vi "Create Commands.vi"(5 "Sequencer":refnum<class "MessageQ.lvclass">, 6 "Variables":refnum<class "Variables.lvclass">, 7 "VolatusAPI":refnum<class "VolatusAPI.lvclass">, 8 "error in (no error)":refnum<class "MultiErrors.lvclass">, 10 "Command Config":refnum<class "Command Config.lvclass">) -> (0 "error out":refnum<class "MultiErrors.lvclass">, 3 "Command":T1)   [LabVIEW 2023, in "VolatusSeq.lvlib" / "State.lvclass"]
uses:
  State.lvclass
  VolatusErrorUtilities/MultiErrors/MultiErrors.lvclass
  VolatusSeqConfig/Command Config/Command Config.lvclass
  Volatus/VolatusAPI/VolatusAPI.lvclass
  Command.ctl
  Volatus/MessageQ/MessageQ.lvclass
  Format String/Format String.lvclass
  VolatusSeqConfig/Command Type.ctl
  messages/CmdDigital/Data.ctl
  messages/CmdAnalog/Data.ctl
  Send Type.ctl
  lv-vecto/Vecto/Channel DBL/Channel DBL.lvclass
  Variables/Variables.lvclass
  VolatusSeqConfig/Digital Command Config/Digital Command Config.lvclass
  VolatusSeqConfig/Numeric Command Config/Numeric Command Config.lvclass
  VolatusSeqConfig/Transition Command Config/Transition Command Config.lvclass
  VolatusSeqConfig/Start Log Command Config/Start Log Command Config.lvclass
  VolatusSeqConfig/Start Seq Command Config/Start Seq Command Config.lvclass
  VolatusSeqConfig/Event Command Config/Event Command Config.lvclass
  VolatusSeqConfig/Error Command Config/Error Command Config.lvclass
  VolatusSeqConfig/HTTP Command Config/HTTP Command Config.lvclass
  VolatusSeqConfig/Reset Var Command Config/Reset Var Command Config.lvclass
  Variables/Variables.lvclass/Variables.ctl
  VolatusSeqConfig/Inc Var Command Config/Inc Var Command Config.lvclass
  VolatusSeqConfig/Dec Var Command Config/Dec Var Command Config.lvclass
  VolatusSeqConfig/Save Var Command Config/Save Var Command Config.lvclass
  VolatusSeqConfig/Load Var Command Config/Load Var Command Config.lvclass
  VolatusSeqConfig/Set Var Command Config/Set Var Command Config.lvclass
  VolatusSeqConfig/Add To Var Command Config/Add To Var Command Config.lvclass
  State.lvclass/State.ctl
  VolatusSeqConfig/VolatusSeqConfig.lvlib
  messages/CmdDigital/CmdDigital.lvlib
  messages/CmdAnalog/CmdAnalog.lvlib
  VolatusSeq.lvlib
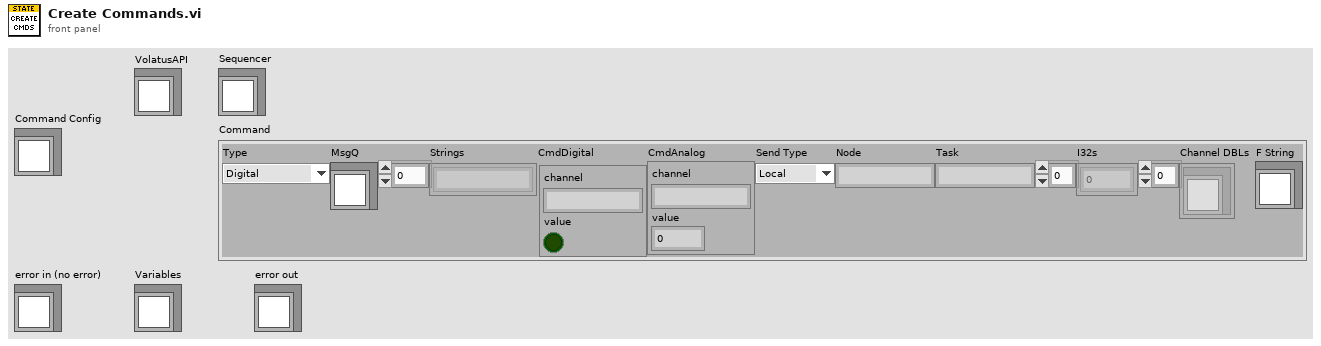
[diagram p1: front panel]
types:
  T1 = typedef "VolatusSeq.lvlib/Command.ctl" = cluster{"Type":T2, "MsgQ":refnum<class "MessageQ.lvclass">, "Strings":string[], "CmdDigital":T3, "CmdAnalog":T4, "Send Type":T5, "Node":string, "Task":string, "I32s":i32[], "Channel DBLs":refnum<class "Channel DBL.lvclass">[], "F String":refnum<class "Format String.lvclass">}
  T2 = typedef "VolatusSeqConfig.lvlib/Command Type.ctl" = enum16{"Digital", "Numeric", "Transition", "Stop", "StartLog", "StopLog", "Start", "Event", "Error", "HTTP", "ResetVar", "IncVar", "DecVar", "SaveVar", "LoadVar", "AddVar", "SubVar", "SetVar", "AddToVar"}
  T3 = typedef "CmdDigital.lvlib/Data.ctl" = cluster{"channel":string, "value":bool}
  T4 = typedef "CmdAnalog.lvlib/Data.ctl" = cluster{"channel":string, "value":dbl}
  T5 = typedef "VolatusSeq.lvlib/Send Type.ctl" = enum16{"Local", "Remote"}
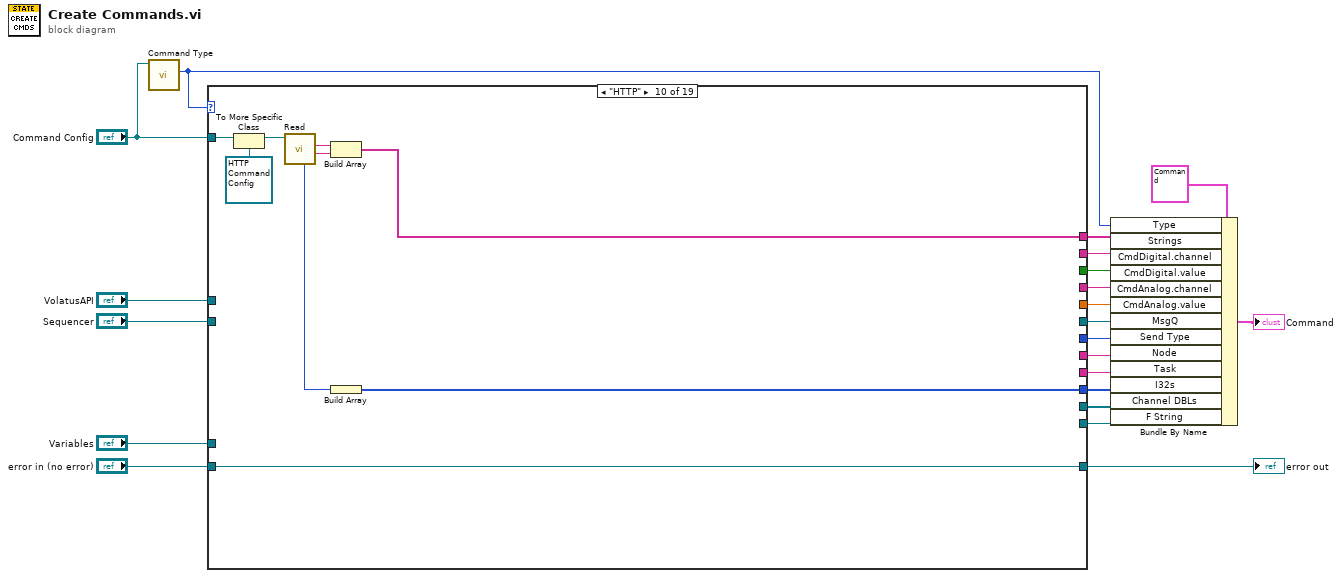
[diagram p0: block diagram]
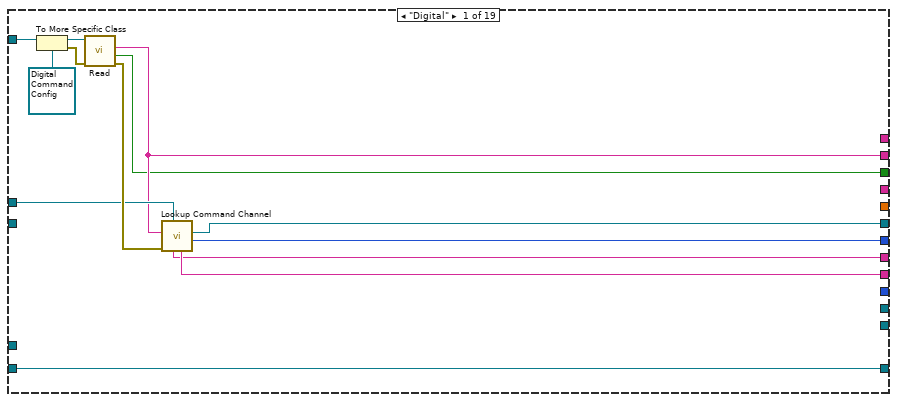
[diagram p2: hidden frame]
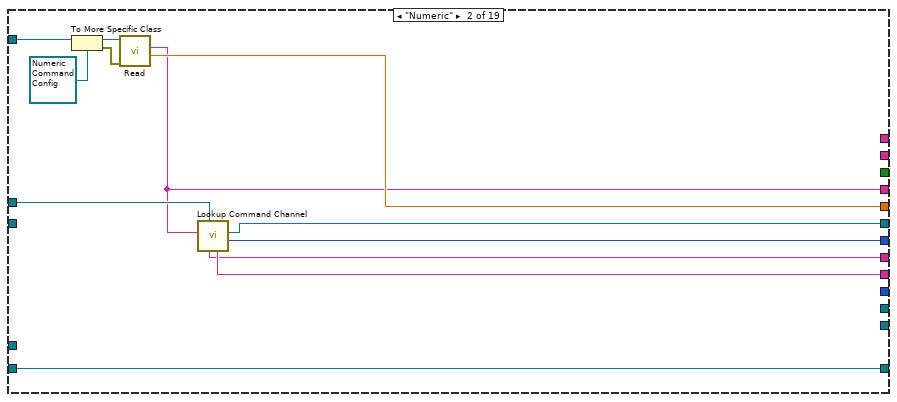
[diagram p3: hidden frame]
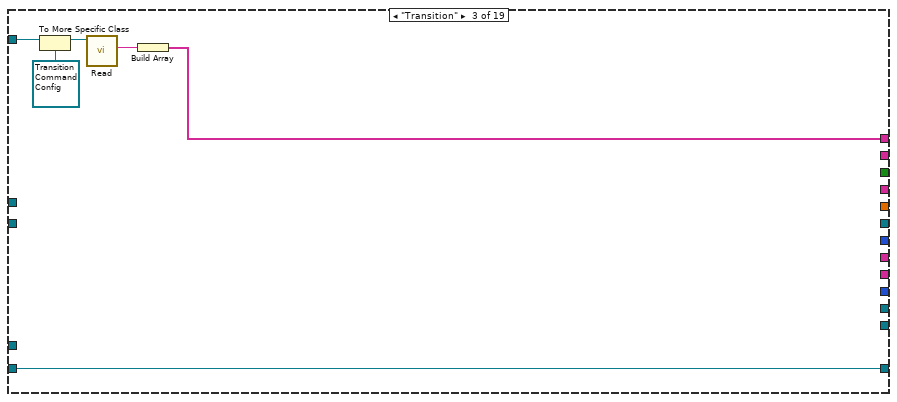
[diagram p4: hidden frame]
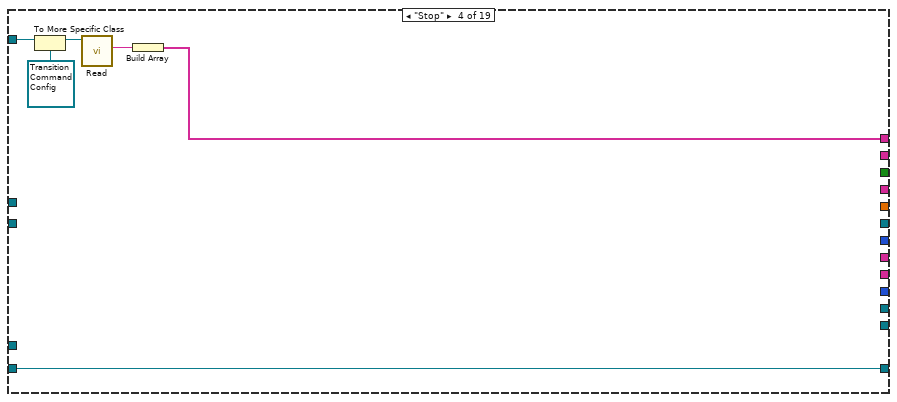
[diagram p5: hidden frame]
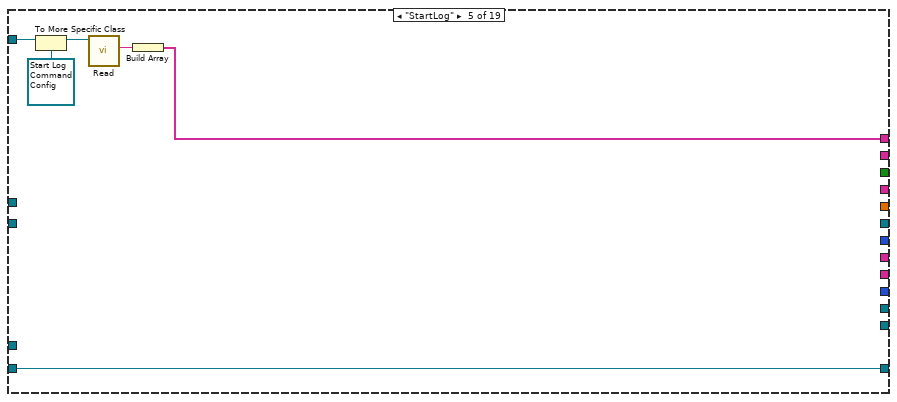
[diagram p6: hidden frame]
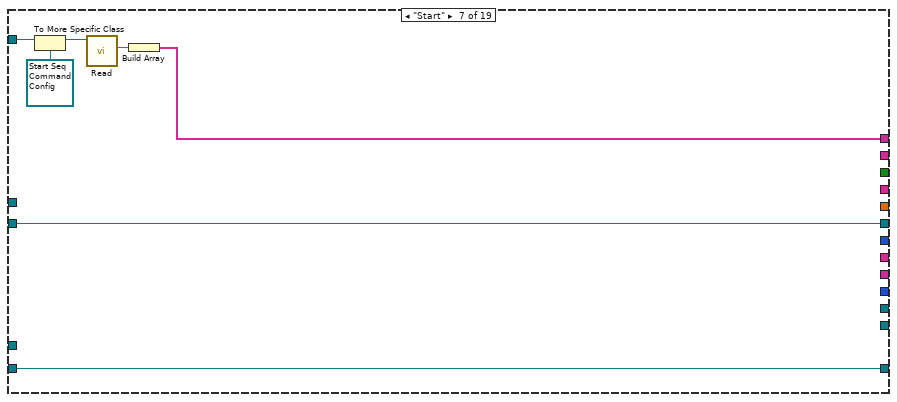
[diagram p8: hidden frame]
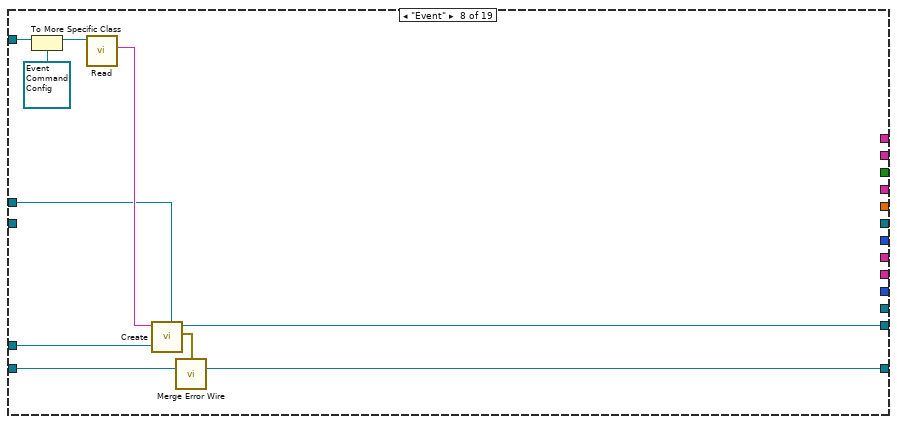
[diagram p9: hidden frame]
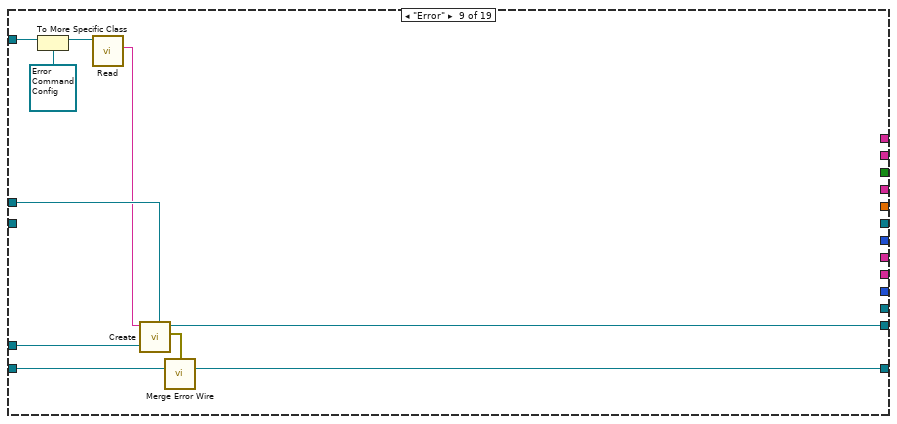
[diagram p10: hidden frame]
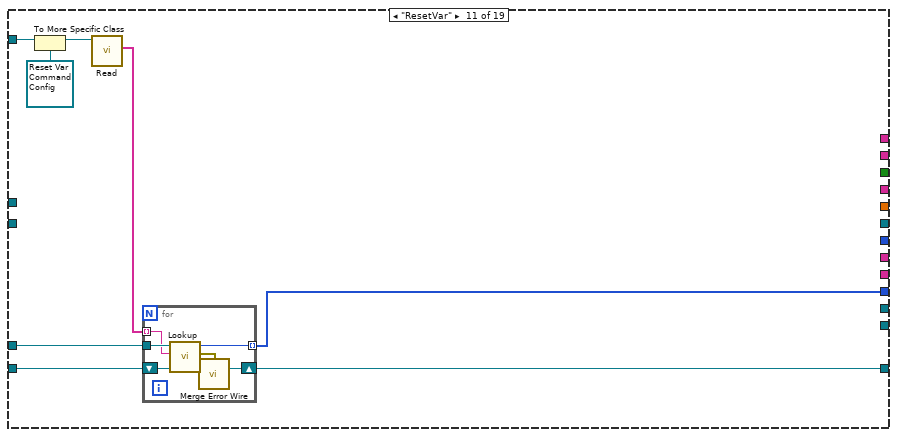
[diagram p11: hidden frame]
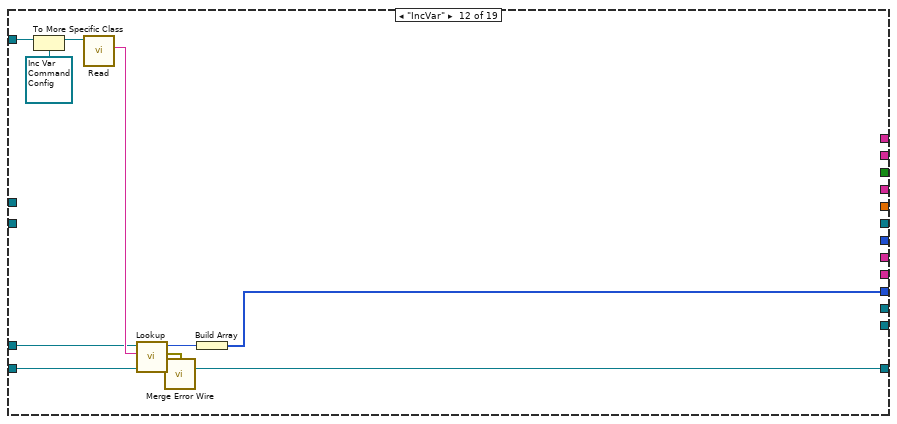
[diagram p12: hidden frame]
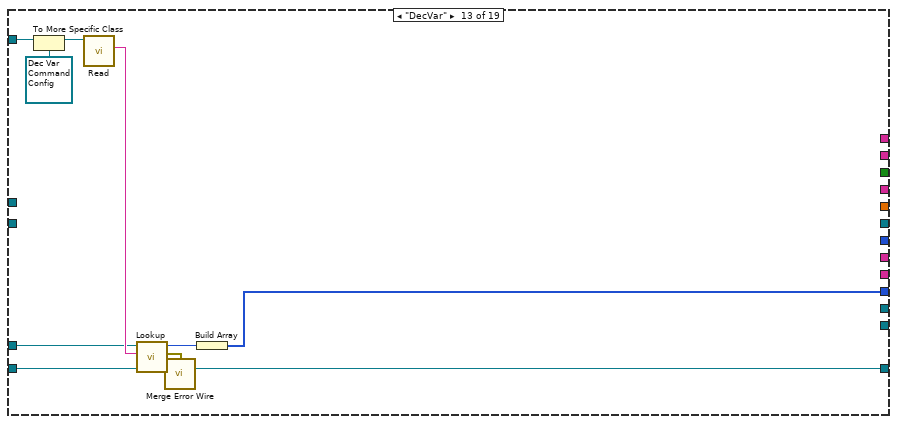
[diagram p13: hidden frame]
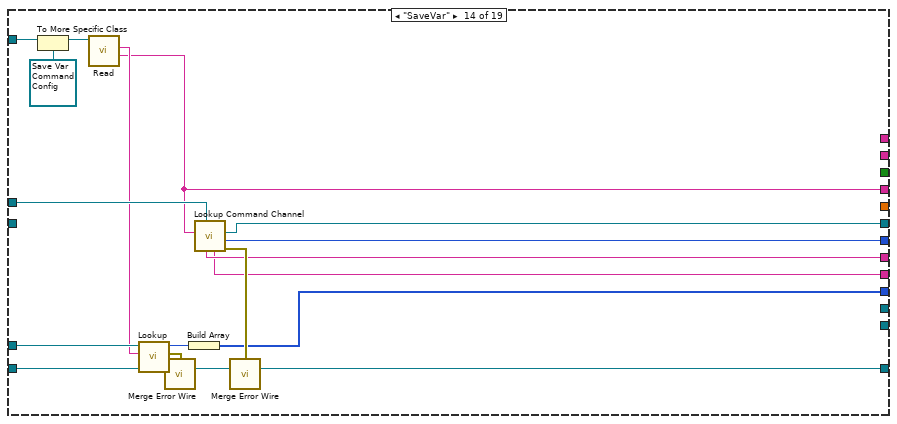
[diagram p14: hidden frame]
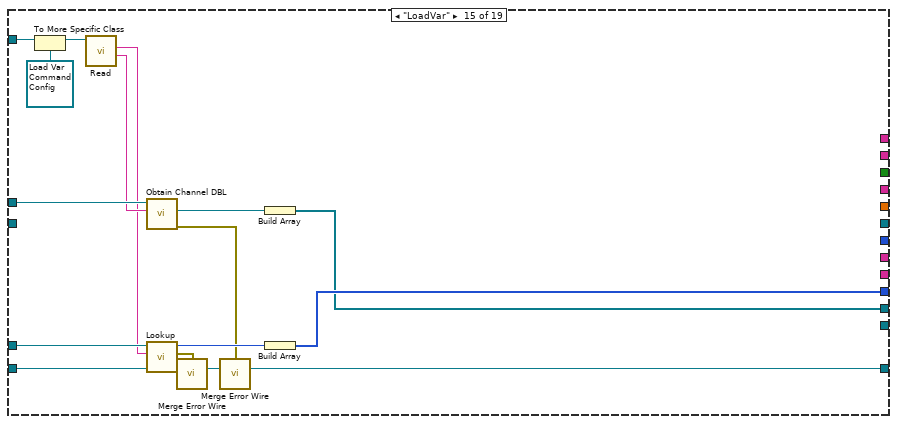
[diagram p15: hidden frame]
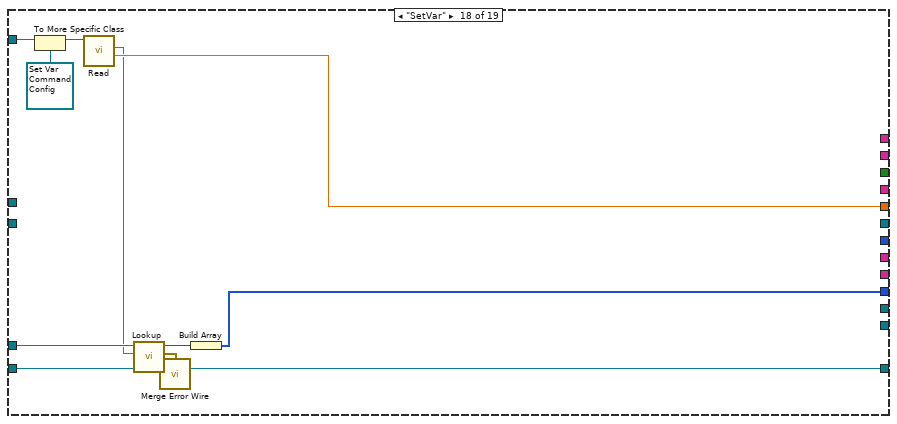
[diagram p18: hidden frame]
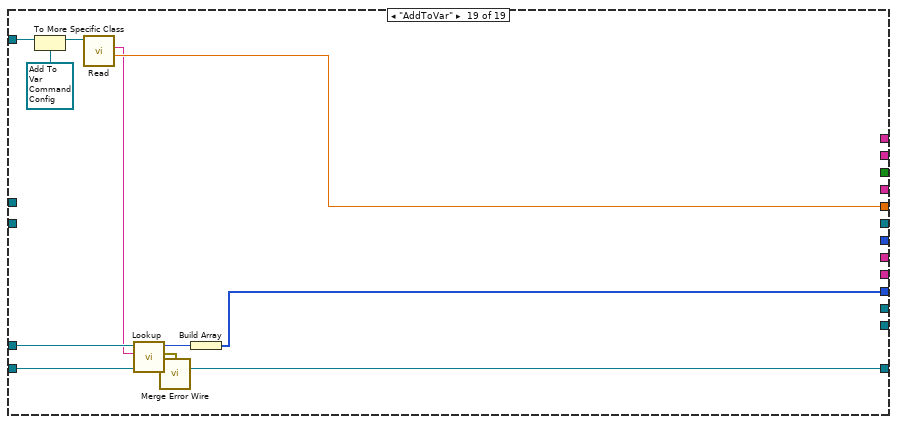
[diagram p19: hidden frame]
diagram:
  n1 = call-dynamic "Command Type.vi"("Command Config in"="Command Config") -> ("Command Type"=w15:T2)  [unwired: 10 in]
  n2 = case shown="\"HTTP\"" w15 {
    tunnel: "Sequencer" -> [_ _ _ _ _ _ w66 _ _ _ _ _ _ _ _ _ _ _ _]
    tunnel: "VolatusAPI" -> [w27 w40 _ _ _ _ _ w76 w87 _ _ _ _ w148 w165 _ _ _ _]
    tunnel: "Variables" -> [_ _ _ _ _ _ _ w77 w88 _ w105 w119 w129 w144 w163 _ _ w177 w188]
    tunnel: "Command Config" -> [w29 w42 w48 w54 w60 _ w68 w79 w89 w96 w106 w120 w130 w151 w168 _ _ w181 w192]
    tunnel: [w34 w46 w52 w58 w64 w65 w72 w74 w84 w101 w104 w118 w128 w138 w155 w170 w171 w173 w184] -> w14
    tunnel: "error in (no error)" -> [w34 w46 w52 w58 w64 w65 w72 w82 w92 w101 w103 w125 w135 w152 w169 w170 w171 w182 w193]
    tunnel: [_ w41 _ _ _ _ _ _ _ _ _ _ _ _ _ _ _ w178 w189] -> w12
    tunnel: [w28 w39 _ _ _ _ _ _ _ _ _ _ _ w137 _ _ _ _ _] -> w11
    tunnel: [w25 w38 _ _ _ _ _ _ _ _ _ _ _ w146 _ _ _ _ _] -> w10
    tunnel: [w24 w37 _ _ _ _ _ _ _ _ _ _ _ w147 _ _ _ _ _] -> w9
    tunnel: [w26 w36 _ _ _ _ w66 _ _ _ _ _ _ w145 _ _ _ _ _] -> w8
    tunnel: [_ w35 _ _ _ _ _ _ _ _ _ _ _ w136 _ _ _ _ _] -> w7
    tunnel: [w23 _ _ _ _ _ _ _ _ _ _ _ _ _ _ _ _ _ _] -> w6
    tunnel: [w22 _ _ _ _ _ _ _ _ _ _ _ _ _ _ _ _ _ _] -> w5
    tunnel: [_ _ w47 w53 w59 _ w67 _ _ w95 _ _ _ _ _ _ _ _ _] -> w4
    tunnel: [_ _ _ _ _ _ _ _ _ w93 w102 w116 w126 w141 w159 _ _ w174 w185] -> w3
    tunnel: [_ _ _ _ _ _ _ _ _ _ _ _ _ _ w158 _ _ _ _] -> w2
    tunnel: [_ _ _ _ _ _ _ w75 w85 _ _ _ _ _ _ _ _ _ _] -> w1
    frame "Digital" {
      n3 = To More Specific Class(target class=refnum<class "Digital Command Config.lvclass"> refnum ("VolatusSeqConfig.lvlib:Digital Command Config.lvclass"), reference=w29) -> (specific class reference=w31:refnum<class "Digital Command Config.lvclass">, error out=w30:errorcluster)  [unwired: 1 in]
      n4 = call "Read.vi"("error in (no error)"=w30, "Digital Command Config in"=w31) -> ("error out"=w33:errorcluster, "Command"=w22:bool, "Channel"=w23:string)  [unwired: 6 in, 1 out]
      n5 = call "Lookup Command Channel.vi"("VolatusAPI in"=w27, "error in (no error)"=w33, "Channel Name"=w23) -> ("Send Type"=w28:T5, "MsgQ"=w26:refnum<class "MessageQ.lvclass">, "Owning Task"=w25:string, "Owning Node"=w24:string)  [unwired: 4 in, 1 out]
    }
    frame "Numeric" {
      n6 = To More Specific Class(target class=refnum<class "Numeric Command Config.lvclass"> refnum ("VolatusSeqConfig.lvlib:Numeric Command Config.lvclass"), reference=w42) -> (specific class reference=w44:refnum<class "Numeric Command Config.lvclass">, error out=w43:errorcluster)  [unwired: 1 in]
      n7 = call "Read.vi"("error in (no error)"=w43, "Numeric Command Config in"=w44) -> ("Command"=w41:dbl, "Channel"=w35:string)  [unwired: 6 in, 2 out]
      n8 = call "Lookup Command Channel.vi"("VolatusAPI in"=w40, "Channel Name"=w35) -> ("Send Type"=w39:T5, "MsgQ"=w36:refnum<class "MessageQ.lvclass">, "Owning Task"=w38:string, "Owning Node"=w37:string)  [unwired: 5 in, 1 out]
    }
    frame "Transition" {
      n9 = To More Specific Class(target class=refnum<class "Transition Command Config.lvclass"> refnum ("VolatusSeqConfig.lvlib:Transition Command Config.lvclass"), reference=w48) -> (specific class reference=w50:refnum<class "Transition Command Config.lvclass">)  [unwired: 1 in, 1 out]
      n10 = call "Read.vi"("Transition Command Config in"=w50) -> ("Target"=w49:string)  [unwired: 8 in, 2 out]
      n11 = Build Array(w49) -> (w47:string[])
    }
    frame "Stop" {
      n12 = To More Specific Class(target class=refnum<class "Transition Command Config.lvclass"> refnum ("VolatusSeqConfig.lvlib:Transition Command Config.lvclass"), reference=w54) -> (specific class reference=w56:refnum<class "Transition Command Config.lvclass">)  [unwired: 1 in, 1 out]
      n13 = call "Read.vi"("Transition Command Config in"=w56) -> ("Target"=w55:string)  [unwired: 8 in, 2 out]
      n14 = Build Array(w55) -> (w53:string[])
    }
    frame "StartLog" {
      n15 = To More Specific Class(target class=refnum<class "Start Log Command Config.lvclass"> refnum ("VolatusSeqConfig.lvlib:Start Log Command Config.lvclass"), reference=w60) -> (specific class reference=w62:refnum<class "Start Log Command Config.lvclass">)  [unwired: 1 in, 1 out]
      n16 = call "Read.vi"("Start Log Command Config in"=w62) -> ("Test"=w61:string)  [unwired: 8 in, 2 out]
      n17 = Build Array(w61) -> (w59:string[])
    }
    frame "StopLog" {
    }
    frame "Start" {
      n18 = To More Specific Class(target class=refnum<class "Start Seq Command Config.lvclass"> refnum ("VolatusSeqConfig.lvlib:Start Seq Command Config.lvclass"), reference=w68) -> (specific class reference=w71:refnum<class "Start Seq Command Config.lvclass">)  [unwired: 1 in, 1 out]
      n19 = call "Read.vi"("Start Seq Command Config in"=w71) -> ("Sequence"=w70:string)  [unwired: 8 in, 2 out]
      n20 = Build Array(w70) -> (w67:string[])
    }
    frame "Event" {
      n21 = To More Specific Class(target class=refnum<class "Event Command Config.lvclass"> refnum ("VolatusSeqConfig.lvlib:Event Command Config.lvclass"), reference=w79) -> (specific class reference=w80:refnum<class "Event Command Config.lvclass">)  [unwired: 1 in, 1 out]
      n22 = call "Read.vi"("Event Command Config in"=w80) -> ("Message"=w78:string)  [unwired: 8 in, 2 out]
      n23 = call "Create.vi"("VolatusAPI"=w76, "Variables"=w77, "F String"=w78) -> ("error out"=w73:errorcluster, "Format String out"=w75:refnum<class "Format String.lvclass">)  [unwired: 7 in]
      n24 = call "Merge Error Wire.vi"("error in (no error)"=w73, "MultiErrors in"=w82) -> ("MultiErrors out"=w74:refnum<class "MultiErrors.lvclass">)  [unwired: 13 in]
    }
    frame "Error" {
      n25 = To More Specific Class(target class=refnum<class "Error Command Config.lvclass"> refnum ("VolatusSeqConfig.lvlib:Error Command Config.lvclass"), reference=w89) -> (specific class reference=w90:refnum<class "Error Command Config.lvclass">)  [unwired: 1 in, 1 out]
      n26 = call "Read.vi"("Error Command Config in"=w90) -> ("Message"=w86:string)  [unwired: 8 in, 2 out]
      n27 = call "Create.vi"("VolatusAPI"=w87, "Variables"=w88, "F String"=w86) -> ("error out"=w83:errorcluster, "Format String out"=w85:refnum<class "Format String.lvclass">)  [unwired: 7 in]
      n28 = call "Merge Error Wire.vi"("error in (no error)"=w83, "MultiErrors in"=w92) -> ("MultiErrors out"=w84:refnum<class "MultiErrors.lvclass">)  [unwired: 13 in]
    }
    frame "HTTP" {
      n29 = To More Specific Class(target class=refnum<class "HTTP Command Config.lvclass"> refnum ("VolatusSeqConfig.lvlib:HTTP Command Config.lvclass"), reference=w96) -> (specific class reference=w99:refnum<class "HTTP Command Config.lvclass">)  [unwired: 1 in, 1 out]
      n30 = call "Read.vi"("HTTP Command Config in"=w99) -> ("Payload"=w97:string, "URL"=w98:string, "Timeout"=w94:i32)  [unwired: 6 in, 2 out]
      n31 = Build Array(w98, w97) -> (w95:string[])
      n32 = Build Array(w94) -> (w93:i32[])
    }
    frame "ResetVar" {
      n33 = To More Specific Class(target class=refnum<class "Reset Var Command Config.lvclass"> refnum ("VolatusSeqConfig.lvlib:Reset Var Command Config.lvclass"), reference=w106) -> (specific class reference=w108:refnum<class "Reset Var Command Config.lvclass">)  [unwired: 1 in, 1 out]
      n34 = call "Read.vi"("Reset Var Command Config in"=w108) -> ("Names"=w107:string[])  [unwired: 8 in, 2 out]
      n35 = for {
        shift-right: [w111] -> w104
        shift-left: w103 -> [w112]
        tunnel: w107 -> [w114] mode=indexing
        tunnel: w105 -> [w115]
        tunnel: [w113] -> w102 mode=indexing
        n36 = call "Lookup.vi"("Name"=w114, "Variables in"=w115) -> ("error out"=w110:errorcluster, "Index"=w113:i32)  [unwired: 8 in]
        n37 = call "Merge Error Wire.vi"("error in (no error)"=w110, "MultiErrors in"=w112) -> ("MultiErrors out"=w111:refnum<class "MultiErrors.lvclass">)  [unwired: 13 in]
      }
    }
    frame "IncVar" {
      n38 = To More Specific Class(target class=refnum<class "Inc Var Command Config.lvclass"> refnum ("VolatusSeqConfig.lvlib:Inc Var Command Config.lvclass"), reference=w120) -> (specific class reference=w124:refnum<class "Inc Var Command Config.lvclass">)  [unwired: 1 in, 1 out]
      n39 = call "Read.vi"("Inc Var Command Config in"=w124) -> ("Name"=w123:string)  [unwired: 8 in, 2 out]
      n40 = call "Lookup.vi"("Name"=w123, "Variables in"=w119) -> ("error out"=w117:errorcluster, "Index"=w122:i32)  [unwired: 8 in]
      n41 = call "Merge Error Wire.vi"("error in (no error)"=w117, "MultiErrors in"=w125) -> ("MultiErrors out"=w118:refnum<class "MultiErrors.lvclass">)  [unwired: 13 in]
      n42 = Build Array(w122) -> (w116:i32[])
    }
    frame "DecVar" {
      n43 = To More Specific Class(target class=refnum<class "Dec Var Command Config.lvclass"> refnum ("VolatusSeqConfig.lvlib:Dec Var Command Config.lvclass"), reference=w130) -> (specific class reference=w134:refnum<class "Dec Var Command Config.lvclass">)  [unwired: 1 in, 1 out]
      n44 = call "Read.vi"("Inc Var Command Config in"=w134) -> ("Name"=w133:string)  [unwired: 8 in, 2 out]
      n45 = call "Lookup.vi"("Name"=w133, "Variables in"=w129) -> ("error out"=w127:errorcluster, "Index"=w132:i32)  [unwired: 8 in]
      n46 = call "Merge Error Wire.vi"("error in (no error)"=w127, "MultiErrors in"=w135) -> ("MultiErrors out"=w128:refnum<class "MultiErrors.lvclass">)  [unwired: 13 in]
      n47 = Build Array(w132) -> (w126:i32[])
    }
    frame "SaveVar" {
      n48 = To More Specific Class(target class=refnum<class "Save Var Command Config.lvclass"> refnum ("VolatusSeqConfig.lvlib:Save Var Command Config.lvclass"), reference=w151) -> (specific class reference=w149:refnum<class "Save Var Command Config.lvclass">)  [unwired: 1 in, 1 out]
      n49 = call "Read.vi"("Save Var Command Config in"=w149) -> ("Channel Name"=w136:string, "Var Name"=w143:string)  [unwired: 7 in, 2 out]
      n50 = call "Lookup.vi"("Name"=w143, "Variables in"=w144) -> ("error out"=w139:errorcluster, "Index"=w142:i32)  [unwired: 8 in]
      n51 = call "Merge Error Wire.vi"("error in (no error)"=w139, "MultiErrors in"=w152) -> ("MultiErrors out"=w140:refnum<class "MultiErrors.lvclass">)  [unwired: 13 in]
      n52 = Build Array(w142) -> (w141:i32[])
      n53 = call "Lookup Command Channel.vi"("VolatusAPI in"=w148, "Channel Name"=w136) -> ("error out"=w153:errorcluster, "Send Type"=w137:T5, "MsgQ"=w145:refnum<class "MessageQ.lvclass">, "Owning Task"=w146:string, "Owning Node"=w147:string)  [unwired: 5 in]
      n54 = call "Merge Error Wire.vi"("error in (no error)"=w153, "MultiErrors in"=w140) -> ("MultiErrors out"=w138:refnum<class "MultiErrors.lvclass">)  [unwired: 13 in]
    }
    frame "LoadVar" {
      n55 = To More Specific Class(target class=refnum<class "Load Var Command Config.lvclass"> refnum ("VolatusSeqConfig.lvlib:Load Var Command Config.lvclass"), reference=w168) -> (specific class reference=w166:refnum<class "Load Var Command Config.lvclass">)  [unwired: 1 in, 1 out]
      n56 = call "Read.vi"("Save Var Command Config in"=w166) -> ("Channel Name"=w164:string, "Var Name"=w162:string)  [unwired: 7 in, 2 out]
      n57 = call "Obtain Channel DBL.vi"("Name"=w164, "VolatusAPI in"=w165) -> ("error out"=w154:errorcluster, "Channel DBL"=w161:refnum<class "Channel DBL.lvclass">)  [unwired: 7 in, 1 out]
      n58 = call "Lookup.vi"("Name"=w162, "Variables in"=w163) -> ("error out"=w156:errorcluster, "Index"=w160:i32)  [unwired: 8 in]
      n59 = call "Merge Error Wire.vi"("error in (no error)"=w156, "MultiErrors in"=w169) -> ("MultiErrors out"=w157:refnum<class "MultiErrors.lvclass">)  [unwired: 13 in]
      n60 = call "Merge Error Wire.vi"("error in (no error)"=w154, "MultiErrors in"=w157) -> ("MultiErrors out"=w155:refnum<class "MultiErrors.lvclass">)  [unwired: 13 in]
      n61 = Build Array(w161) -> (w158:refnum<class "Channel DBL.lvclass">[])
      n62 = Build Array(w160) -> (w159:i32[])
    }
    frame "AddVar" {
    }
    frame "SubVar" {
    }
    frame "SetVar" {
      n63 = To More Specific Class(target class=refnum<class "Set Var Command Config.lvclass"> refnum ("VolatusSeqConfig.lvlib:Set Var Command Config.lvclass"), reference=w181) -> (specific class reference=w179:refnum<class "Set Var Command Config.lvclass">)  [unwired: 1 in, 1 out]
      n64 = call "Read.vi"("Set Var Command Config in"=w179) -> ("Value"=w178:dbl, "Var"=w176:string)  [unwired: 7 in, 2 out]
      n65 = call "Lookup.vi"("Name"=w176, "Variables in"=w177) -> ("error out"=w172:errorcluster, "Index"=w175:i32)  [unwired: 8 in]
      n66 = call "Merge Error Wire.vi"("error in (no error)"=w172, "MultiErrors in"=w182) -> ("MultiErrors out"=w173:refnum<class "MultiErrors.lvclass">)  [unwired: 13 in]
      n67 = Build Array(w175) -> (w174:i32[])
    }
    frame "AddToVar" {
      n68 = To More Specific Class(target class=refnum<class "Add To Var Command Config.lvclass"> refnum ("VolatusSeqConfig.lvlib:Add To Var Command Config.lvclass"), reference=w192) -> (specific class reference=w190:refnum<class "Add To Var Command Config.lvclass">)  [unwired: 1 in, 1 out]
      n69 = call "Read.vi"("Add To Var Command Config in"=w190) -> ("Value"=w189:dbl, "Variable"=w187:string)  [unwired: 7 in, 2 out]
      n70 = call "Lookup.vi"("Name"=w187, "Variables in"=w188) -> ("error out"=w183:errorcluster, "Index"=w186:i32)  [unwired: 8 in]
      n71 = call "Merge Error Wire.vi"("error in (no error)"=w183, "MultiErrors in"=w193) -> ("MultiErrors out"=w184:refnum<class "MultiErrors.lvclass">)  [unwired: 13 in]
      n72 = Build Array(w186) -> (w185:i32[])
    }
  }
  "error out" <- w14
  n73 = Bundle By Name(cluster=T1 {"Type"=enum."Digital", "MsgQ"=refnum, "Strings"=[], "CmdDigital"={"channel"="", "value"=FALSE}, "CmdAnalog"={"channel"="", "value"=0.0}, "Send Type"=enum."Local", "Node"="", "Task"="", "I32s"=[], "Channel DBLs"=[], "F String"=refnum} ("Command"), "Type"=w15, "Strings"=w4, "CmdDigital.channel"=w6, "CmdDigital.value"=w5, "CmdAnalog.channel"=w7, "CmdAnalog.value"=w12, "MsgQ"=w8, "Send Type"=w11, "Node"=w9, "Task"=w10, "I32s"=w3, "Channel DBLs"=w2, "F String"=w1) -> (→"Command":T1)
